vi "Example_Kernel PCA.vi"() -> ()   [LabVIEW 2009]
uses:
  <vilib>/Utility/miscctls.llb/LV3DPointTypeDef.ctl
  <vilib>/addons/Machine Learning/Visualization/Visualization (3D).vi
  <vilib>/addons/Machine Learning/NILabs_MLT.lvlib
panel:
  out "3-D Projection of the data":refnum<vi>(3d-picture)
  in  "Parameter":dbl=2.0
  in  "Kernel type":T1(ring)=enum."Polynomial Kernel"
  in  "# of circles":i32=2
  out "error out":errorcluster
  in  "# of samples":i32=1024
  out "2-D data":refnum<vi>(3d-picture)
  # "Introduction:\nKernel Principle Component Analysis (PCA) is a non-linear mapping method. For a clustering problem such as this example, an appropriate kernel can help mapping a non-linearly separable data set to a higher-dimensional space where the projection of the data are linearly separable."
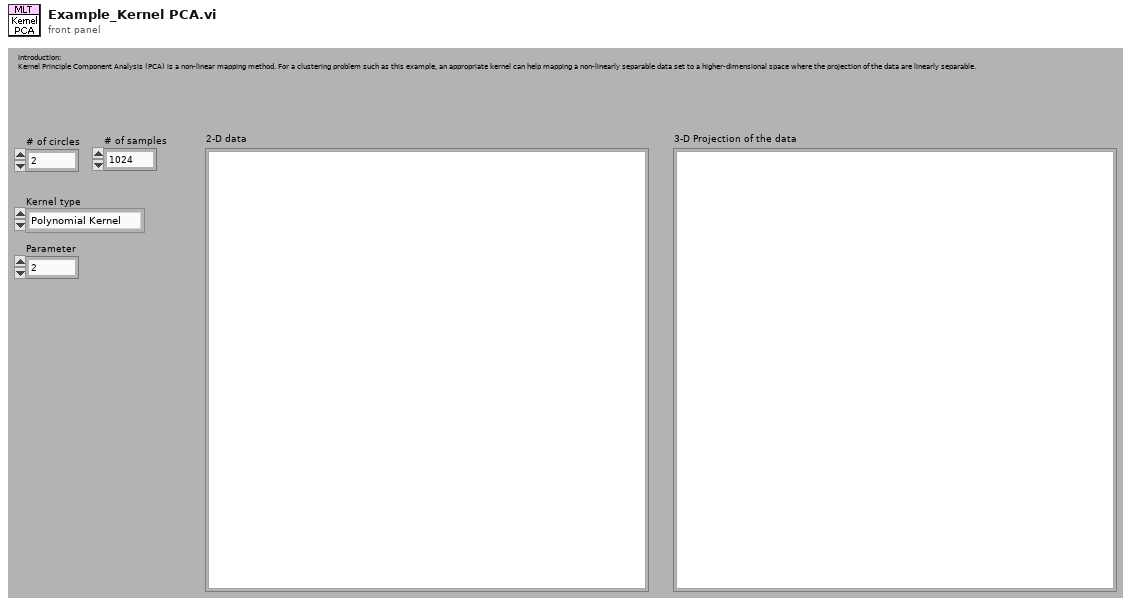
[diagram p1: front panel]
types:
  T1 = enum16{"Linear Kernel", "Polynomial Kernel", "Gaussian Kernel"}
  T2 = typedef "LV3DPointTypeDef.ctl" = cluster{"X":sgl, "Y":sgl, "Z":sgl}
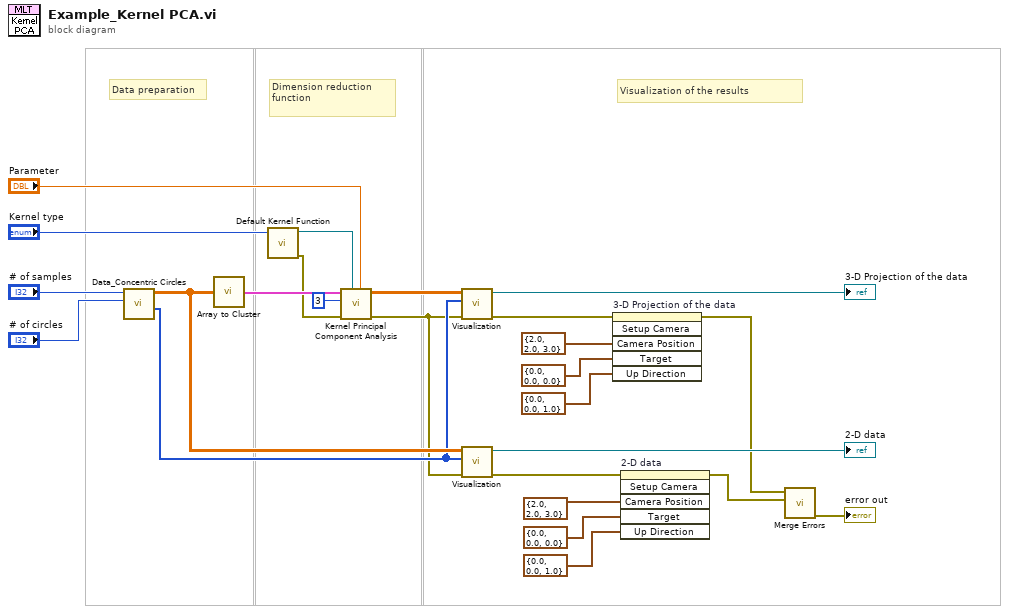
[diagram p0: block diagram]
diagram:
  # "Visualization of the results"
  # "Dimension reduction function"
  # "Data preparation"
  n1 = call "Data_Concentric Circles.vi"("# of circles"="# of circles", "# of points"="# of samples") -> ("Classes"=w11:i32[], "Data"=w21:dbl[][])  [unwired: 8 in]
  n2 = call <vilib>:"Array to Cluster.vi"("Data in Array"=w21) -> ("Data in Cluster"=w19:cluster{"Sample":dbl[]}[])
  n3 = call <vilib>:"Default Kernel Function.vi"("kernel type"="Kernel type") -> ("error out"=w3:errorcluster, "Kernel Function"=w15:refnum<vi>)  [unwired: 9 in]
  n4 = call <vilib>:"Kernel Principal Component Analysis.vi"("parameters"="Parameter", "Kernel Function"=w15, "error in (no error)"=w3, "dim"=3, "Data samples"=w19) -> ("error out"=w5:errorcluster, "Features"=w18:dbl[][])  [unwired: 3 in, 2 out]
  n5 = call-poly <vilib>:"Visualization.vi"("error in (no error)"=w5, "Class labels"=w11, "Data samples"=w18) -> ("error out"=w6:errorcluster, "3D Picture"=→"3-D Projection of the data":refnum<vi>)  [unwired: 7 in]
  n6 = call-poly <vilib>:"Visualization.vi"("error in (no error)"=w5, "Class labels"=w11, "Data samples"=w21) -> ("error out"=w17:errorcluster, "3D Picture"=→"2-D data":refnum<vi>)  [unwired: 7 in]
  n7 = invoke on="3-D Projection of the data" class="SceneGraphDisp (strict)" method="Setup Camera"(error in=w6, "Camera Position"=T2 {"X"=2.0, "Y"=2.0, "Z"=3.0}, "Target"=T2 {"X"=0.0, "Y"=0.0, "Z"=0.0} ("Camera Position"), "Up Direction"=T2 {"X"=0.0, "Y"=0.0, "Z"=1.0} ("Camera Position")) -> (error out=w2:errorcluster)  [unwired: 2 in, 5 out]
  n8 = invoke on="2-D data" class="SceneGraphDisp (strict)" method="Setup Camera"(error in=w17, "Camera Position"=T2 {"X"=2.0, "Y"=2.0, "Z"=3.0}, "Target"=T2 {"X"=0.0, "Y"=0.0, "Z"=0.0} ("Camera Position"), "Up Direction"=T2 {"X"=0.0, "Y"=0.0, "Z"=1.0} ("Camera Position")) -> (error out=w1:errorcluster)  [unwired: 2 in, 5 out]
  n9 = call <vilib>:"Merge Errors.vi"("error in 2 (no error)"=w1, "error in 1 (no error)"=w2) -> ("error out"=→"error out":errorcluster)  [unwired: 5 in]
